vi "CDEW_SpecPage.vi"(10 "Spec Page Interface":T3, 11 "MetaDataObj in":refnum<class "MetaDataObj.lvclass">) -> (3 "MetaDataObj out":refnum<class "MetaDataObj.lvclass">)   [LabVIEW 2026, in "NIVS_CDEW_MetaDataObj.lvclass"]
uses:
  NIVS_CDEW_MetaDataObj.lvclass
  <resource>/dialog/NewProjectWizard/Spec Page Interface.ctl
  <resource>/dialog/NewProjectWizard/MetaDataObj/MetaDataObj.lvclass
  Types/Execution Modes.ctl
  Types/Wizard Conditional Controls.ctl
  NIVS_CDEW_MetaDataObj.lvclass/NIVS_CDEW_MetaDataObj.ctl
  <resource>/dialog/NewProjectWizard/MetaDataObj/MetaDataObj.lvclass/MetaDataObj.ctl
  <resource>/dialog/NewProjectWizard/MetaDataObj/Accessors/Write Project Name.vi
  <resource>/dialog/NewProjectWizard/MetaDataObj/Accessors/Write Project Root.vi
  C:/Program Files/National Instruments/LabVIEW 2026/resource/dialog/NewProjectWizard/MetaDataObj/MetaDataObj.lvclass
  C:/Program Files/National Instruments/LabVIEW 2026/ProjectTemplates/Source/NI VeriStand/Custom Device Express/Custom Device/NIVS_CDEW_MetaDataObj/NIVS_CDEW_MetaDataObj.lvclass
panel:
  out "error out":errorcluster
  out "Warning":string="*LabVIEW RT not installed, Linux_x64 disabled!"
  in  "Custom Device Target OS":enum16{"Linux_x64", "Windows", "All"}(ring)
  in  "Operation":T1(ring)
  in  "LaunchXMLEditor":bool
  in  "Custom Device Execution Mode":T2
  in  "Custom Device Name":string
  in  "Custom Device Root Folder":path=path "<specify path>"
  in  "Custom Device XML File":path=path "<specify path>"
  in  "Retain .Net APIs":bool
  in  "Retain LV Projects":bool
  in  "Parent Menu Name":string="National Instruments"
  in  "Submenu":bool
  in  "Maximum Custom Device Instances":i32=1 min=1 max=2474 step=1
  # "Advanced Options"
  # "Insert Custom Device in Submenu"
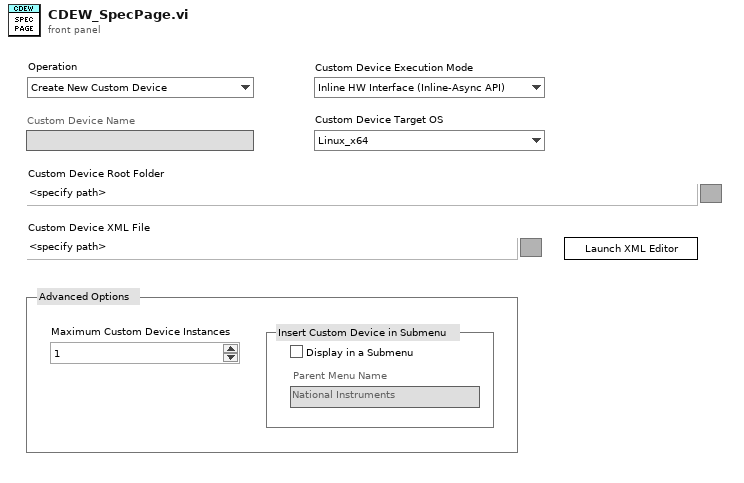
[diagram p1: front panel]
types:
  T1 = enum16{"Create New Custom Device", "Edit Existing Custom Device"}
  T2 = typedef "NIVS_CDEW_MetaDataObj.lvclass/Execution Modes.ctl" = enum16{"Inline HW Interface (Inline-Async API)", "Inline HW Interface"}
  T3 = typedef "Spec Page Interface.ctl" = cluster{"\"Tab Forward To\" Refnum":refnum<vi>, "\"Tab Backward To\" Refnum":refnum<vi>, "Errors":refnum<user-event>, "Quit":refnum<user-event>}
  T4 = typedef "NIVS_CDEW_MetaDataObj.lvclass/Wizard Conditional Controls.ctl" = cluster{"XML File Path":refnum<vi>, "Submenu":refnum<vi>, "Parent Menu Name":refnum<vi>, "Retain .Net APIs":refnum<vi>, "User Action":refnum<vi>, "Execution Mode":refnum<vi>}
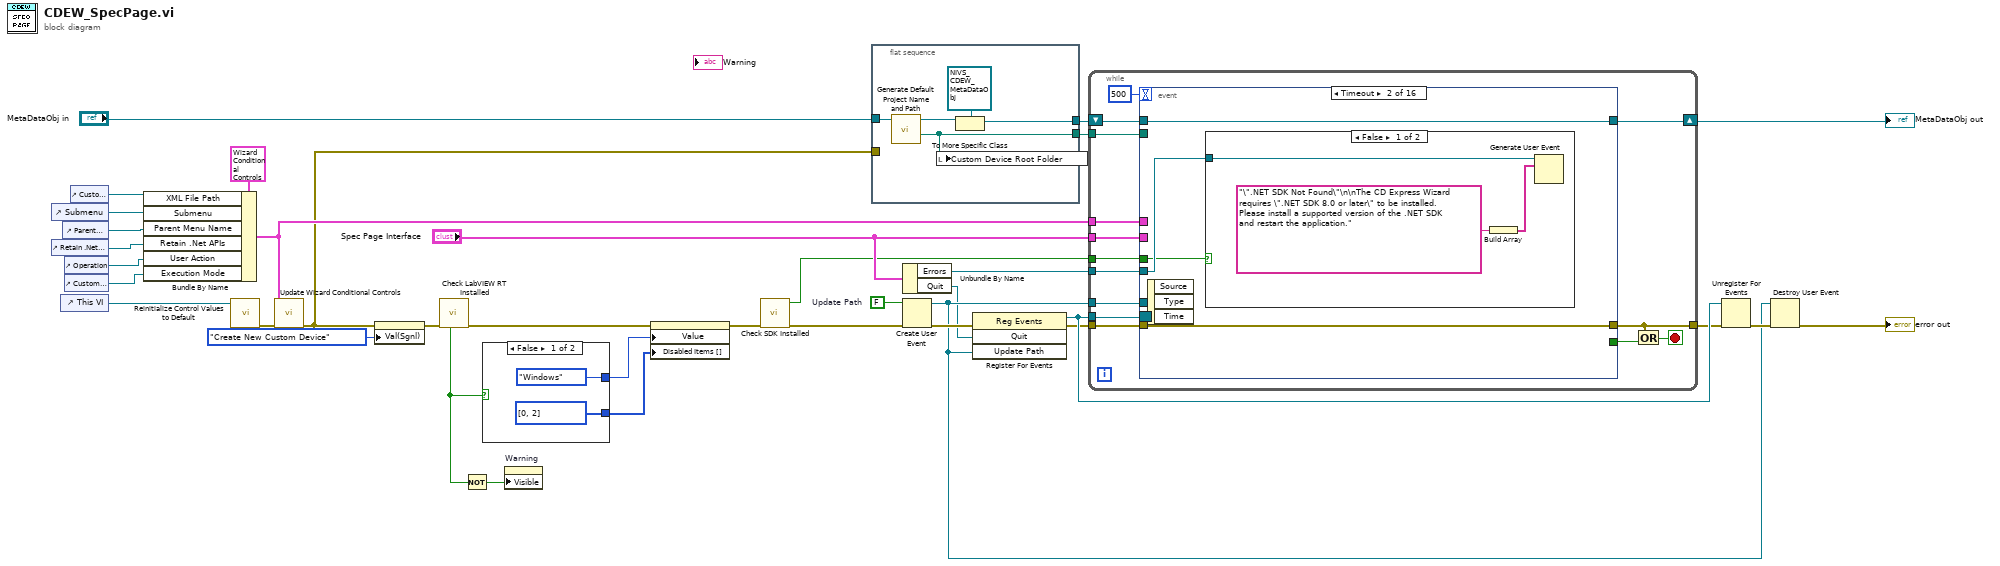
[diagram p0: block diagram]
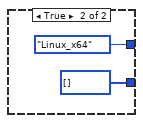
[diagram p2: hidden frame]
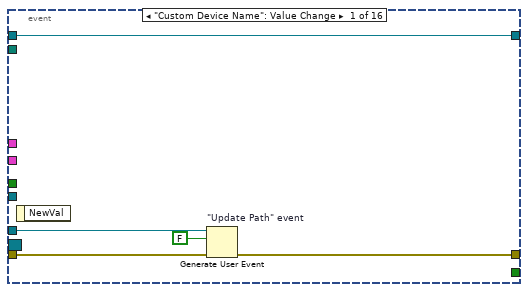
[diagram p3: hidden frame]
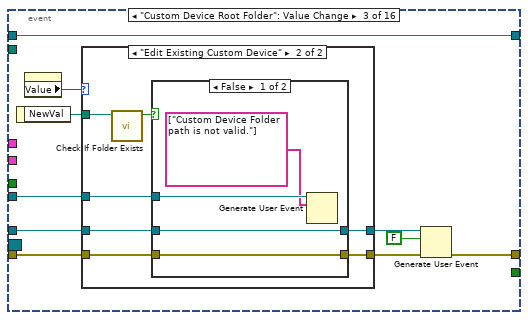
[diagram p5: hidden frame]
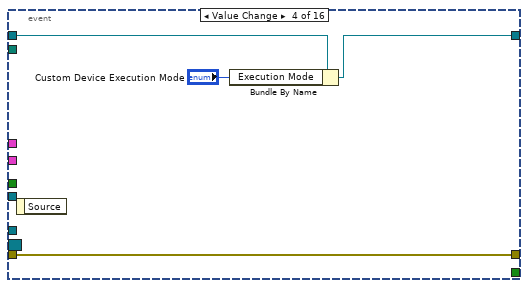
[diagram p8: hidden frame]
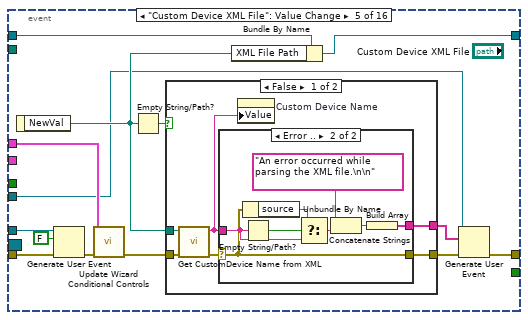
[diagram p9: hidden frame]
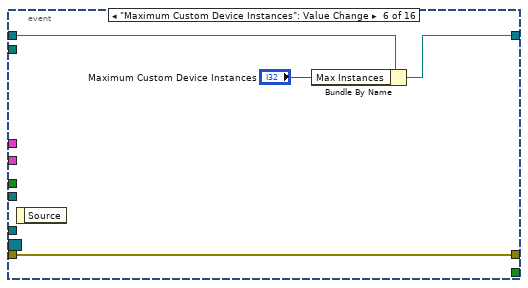
[diagram p12: hidden frame]
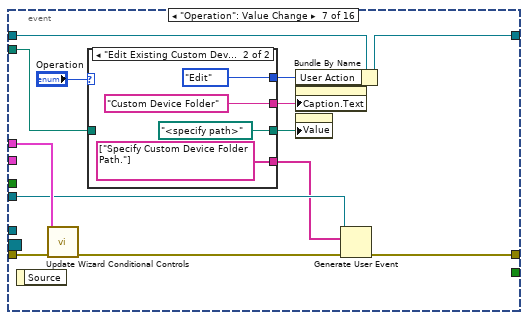
[diagram p13: hidden frame]
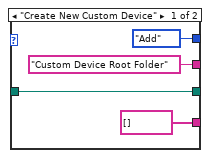
[diagram p14: hidden frame]
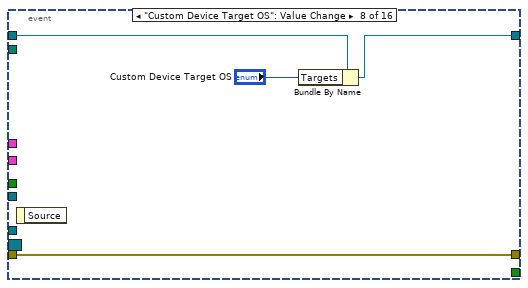
[diagram p15: hidden frame]
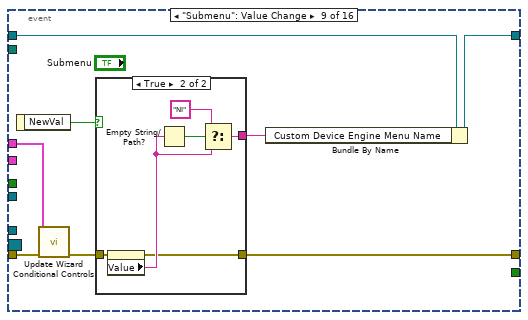
[diagram p16: hidden frame]
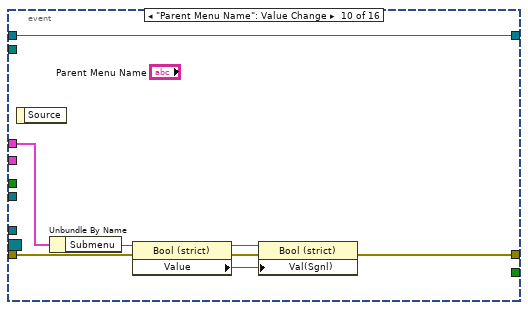
[diagram p18: hidden frame]
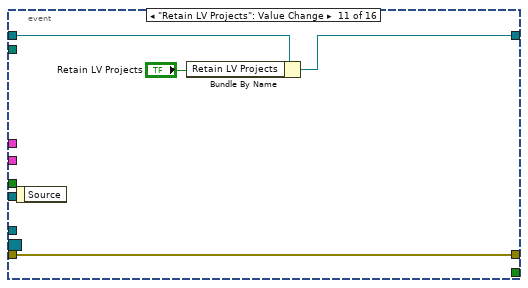
[diagram p19: hidden frame]
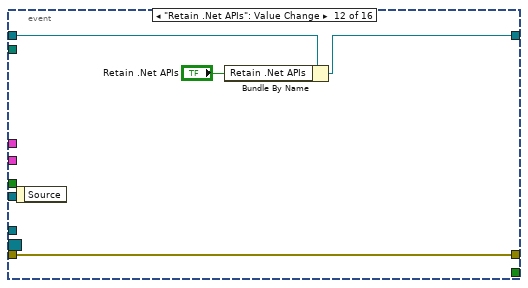
[diagram p20: hidden frame]
diagram:
  w19 = FALSE  # Update Path
  n1 = control-ref of="Submenu"() -> (w32:refnum<vi>)
  n2 = control-ref of="Retain .Net APIs"() -> (w34:refnum<vi>)
  n3 = control-ref of="This VI"() -> (w35:refnum<vi>)
  n4 = control-ref of="Parent Menu Name"() -> (w33:refnum<vi>)
  n5 = control-ref of="Operation"() -> (w25:refnum<vi>)
  n6 = control-ref of="Custom Device Execution Mode"() -> (w26:refnum<vi>)
  n7 = control-ref of="Custom Device XML File"() -> (w31:refnum<vi>)
  n8 = Bundle By Name(cluster=T4 {"XML File Path"=refnum, "Submenu"=refnum, "Parent Menu Name"=refnum, "Retain .Net APIs"=refnum, "User Action"=refnum, "Execution Mode"=refnum} ("Wizard_ConditionalControls"), "XML File Path"=w31, "Submenu"=w32, "Parent Menu Name"=w33, "Retain .Net APIs"=w34, "User Action"=w25, "Execution Mode"=w26) -> (w36:T4)
  n9 = call "Reinitialize Control Values to Default.vi"("VI Ref"=w35) -> ("error out"=w29:errorcluster)  [unwired: 10 in]
  n10 = call "Update Wizard Conditional Controls.vi"("error in"=w29, "Wizard_Conditional Controls"=w36) -> ("error out"=w24:errorcluster)  [unwired: 9 in]
  n11 = property on="Operation" class="Enum (strict)"(error in=w24, "Val(Sgnl)"=T1."Create New Custom Device" ("Value (Signaling)")) -> (error out=w7:errorcluster)  [unwired: 1 in, 1 out]
  n12 = call "Check LabVIEW RT Installed.vi"("error in"=w7) -> ("error out"=w13:errorcluster, "labview rt installed?"=w10:bool)  [unwired: 5 in, 4 out]
  n13 = Not(x=w10) -> (.not. x?=w9:bool)
  n14 = case shown="False" w10 {
    tunnel: [enum16{"Linux_x64", "Windows", "All"}."Windows" ("Custom Device Target OS") enum16{"Linux_x64", "Windows", "All"}."Linux_x64" ("Custom Device Target OS")] -> w12
    tunnel: [i32[] [0, 2] ("Disabled Items []") i32[] [] ("Disabled Items []")] -> w11
    frame False {
    }
    frame True {
    }
  }
  n15 = property on="Warning" class="Str"("Visible"=w9) -> ()  [unwired: 2 in, 2 out]
  n16 = property on="Custom Device Target OS" class="Enum (strict)"(error in=w13, "Value"=w12, "Disabled Items []"=w11) -> (error out=w3:errorcluster)  [unwired: 1 in, 1 out]
  n17 = call "Check SDK Installed.vi"("error in"=w3) -> ("error out"=w2:errorcluster, ".Net SDK Available?"=w1:bool)  [unwired: 9 in]
  n18 = flat-sequence {
    tunnel: [w44] -> w16
    tunnel: "MetaDataObj in" -> [w43]
    tunnel: w24 -> [_]
    tunnel: [w41] -> w14
    frame #0 {
      n19 = call <resource>:"Generate Default Project Name and Path.vi"("DNL_MetaDataObj in"=w43) -> ("Project Root"=w41:path, "DNL_MetaDataObj out"=w42:refnum<class "MetaDataObj.lvclass">)  [unwired: 8 in, 1 out]
      n20 = local write "Custom Device Root Folder"(w41) -> ()
      n21 = To More Specific Class(target class=refnum<class "NIVS_CDEW_MetaDataObj.lvclass"> refnum ("Consolidated_CD"), reference=w42) -> (specific class reference=w44:refnum<class "NIVS_CDEW_MetaDataObj.lvclass">)  [unwired: 1 in, 1 out]
    }
  }
  n22 = Unbundle By Name("Spec Page Interface") -> ("Errors"=w5:refnum<user-event>, "Quit"=w6:refnum<user-event>)
  n23 = Create User Event(user event datatype=w19, error in=w2) -> (user event=w15:refnum<user-event>, error out=w18:errorcluster)
  n24 = register-events(error in=w18, w6, w15) -> (reference out=w21:refnum<event-registration>, error out=w4:errorcluster)  [unwired: 1 in]
  n25 = while {
    tunnel: "Spec Page Interface" -> [w58]
    shift-right: [w57] -> w28
    shift-left: w16 -> [w56]
    tunnel: w21 -> [w59]
    tunnel: [w53] -> w20
    tunnel: w4 -> [w52]
    tunnel: w15 -> [w51]
    tunnel: w36 -> [w50]
    tunnel: w5 -> [w49]
    tunnel: w14 -> [w48]
    tunnel: w1 -> [w46]
    stop <- w55 stop-if-true
    n26 = event shown="[1] Timeout" {
      selector: w59 -> [_ _ _ _ _ _ _ _ _ _ _ _ _ _ _ _]
      dyn-events: _ -> [_ _ _ _ _ _ _ _ _ _ _ _ _ _ _ _]
      timeout: 500 -> [_ _ _ _ _ _ _ _ _ _ _ _ _ _ _ _]
      tunnel: w58 -> [_ _ _ _ _ _ _ _ _ _ _ _ _ w202 _ _]
      tunnel: [_ _ _ _ _ _ _ _ _ _ _ _ _ _ _ w220] -> w54
      tunnel: [w64 w66 w80 w100 w103 w134 w139 w159 w161 w176 w186 w190 w197 w198 w208 w217] -> w53
      tunnel: [w62 w68 w81 w98 w114 w132 w147 w158 w167 w178 w185 w188 w195 w199 w210 w219] -> w57
      tunnel: w56 -> [w62 w68 w81 w99 w113 w131 w146 w157 w166 w178 w184 w187 w194 w199 w209 w219]
      tunnel: w52 -> [w61 w66 w77 w100 w110 w134 w135 w159 w160 w175 w186 w190 w197 w198 w207 w216]
      tunnel: w51 -> [w60 _ w78 _ w109 _ _ _ _ _ _ _ _ _ _ _]
      tunnel: w50 -> [_ _ _ _ w112 _ w143 _ w163 w182 _ _ w193 _ _ _]
      tunnel: w49 -> [_ w67 w72 _ w102 _ w138 _ _ _ _ _ _ _ _ w218]
      tunnel: w48 -> [_ _ _ _ _ _ w140 _ _ _ _ _ _ _ _ _]
      tunnel: w46 -> [_ w65 _ _ _ _ _ _ _ _ _ _ _ _ _ _]
      event "Custom Device Name": Value Change {
        n27 = event-data() -> ()  [unwired: 1 in, 1 out]
        n28 = Generate User Event "\"Update Path\" event"(user event=w60, event data cluster=FALSE ("event data"), error in=w61) -> (error out=w64:errorcluster)  [unwired: 1 in, 1 out]
      }
      event Timeout {
        n29 = event-data() -> ()  [unwired: 1 in, 3 out]
        n30 = case shown="False" w65 {
          tunnel: w67 -> [w71 _]
          frame False {
            n31 = Build Array("\".NET SDK Not Found\"\n\nThe CD Express Wizard requires \".NET SDK 8.0 or later\" to be installed. Please install a supported version of the .NET SDK and restart the application." ("message")) -> (w69:string[])
            n32 = Generate User Event(user event=w71, event data cluster=w69) -> ()  [unwired: 2 in, 2 out]
          }
          frame True {
          }
        }
      }
      event "Custom Device Root Folder": Value Change {
        n33 = event-data() -> ("NewVal"=w73:path)  [unwired: 1 in]
        n34 = property on="Operation" class="Enum (strict)"() -> ("Value"=w76:T1)  [unwired: 2 in, 2 out]
        n35 = case shown="\"Edit Existing Custom Device\"" w76 {
          tunnel: w78 -> [w82 w88]
          tunnel: w77 -> [w83 w89]
          tunnel: [w83 w85] -> w75
          tunnel: [w82 w84] -> w74
          tunnel: w73 -> [_ w90]
          tunnel: w72 -> [_ w86]
          frame "Create New Custom Device" {
          }
          frame "Edit Existing Custom Device" {
            n36 = call "Check If Folder Exists.vi"("Folder Path"=w90) -> ("Valid Folder?"=w87:bool)  [unwired: 10 in]
            n37 = case shown="False" w87 {
              tunnel: w89 -> [w92 w96]
              tunnel: w88 -> [w93 w95]
              tunnel: w86 -> [w94 _]
              tunnel: [w92 w96] -> w85
              tunnel: [w93 w95] -> w84
              frame False {
                n38 = Generate User Event ("\"Update Path\" event")(user event=w94, event data cluster=string[] ["Custom Device Folder path is not valid."] ("event data")) -> ()  [unwired: 2 in, 2 out]
              }
              frame True {
              }
            }
          }
        }
        n39 = Generate User Event ("\"Update Path\" event")(user event=w74, event data cluster=FALSE ("event data"), error in=w75) -> (error out=w80:errorcluster)  [unwired: 1 in, 1 out]
      }
      event Value Change {
        n40 = event-data() -> ()  [unwired: 1 in, 1 out]
        n41 = Bundle By Name(cluster=w99, "Execution Mode"="Custom Device Execution Mode") -> (w98:refnum<class "NIVS_CDEW_MetaDataObj.lvclass">)
      }
      event "Custom Device XML File": Value Change {
        n42 = event-data() -> ("NewVal"=w105:path)  [unwired: 1 in]
        n43 = Generate User Event ("\"Update Path\" event")(user event=w109, event data cluster=FALSE ("event data"), error in=w110) -> (error out=w108:errorcluster)  [unwired: 1 in, 1 out]
        n44 = call "Update Wizard Conditional Controls.vi"("error in"=w108, "Wizard_Conditional Controls"=w112) -> ("error out"=w107:errorcluster)  [unwired: 9 in]
        n45 = Empty String/Path?(string/path=w105) -> (empty?=w106:bool)
        n46 = case shown="False" w106 {
          tunnel: w107 -> [w120 w130]
          tunnel: w105 -> [w119 _]
          tunnel: [w117 w130] -> w104
          tunnel: [w116 _] -> w101
          frame False {
            n47 = call "Get CustomDevice Name from XML.vi"("error in"=w120, "XML File Path"=w119) -> ("error out"=w118:errorcluster, "Custom Device Name"=w115:string)  [unwired: 8 in]
            n48 = case shown="Error .." w118 {
              selector: w118 -> [w121 w122]
              tunnel: w115 -> [_ w128]
              tunnel: [_ w123] -> w116
              tunnel: [w121 w122] -> w117
              frame No Error {
              }
              frame Error {
                n49 = Unbundle By Name(w122) -> ("source"=w127:string)
                n50 = Empty String/Path?(string/path=w128) -> (empty?=w129:bool)
                n51 = Select(t=w127, s=w129, f=w128) -> (s? t:f=w126:string)
                n52 = Concatenate Strings("An error occurred while parsing the XML file.\n\n" ("string"), w126) -> (w124:string)
                n53 = Build Array(w124) -> (w123:string[])
              }
            }
            n54 = property on="Custom Device Name" class="Str"("Value"=w115) -> ()  [unwired: 2 in, 2 out]
          }
          frame True {
          }
        }
        n55 = Bundle By Name(cluster=w113, "XML File Path"=w105) -> (w114:refnum<class "NIVS_CDEW_MetaDataObj.lvclass">)
        n56 = Generate User Event ("\"Update Path\" event")(user event=w102, event data cluster=w101, error in=w104) -> (error out=w103:errorcluster)  [unwired: 1 in, 1 out]
      }
      event "Maximum Custom Device Instances": Value Change {
        n57 = event-data() -> ()  [unwired: 1 in, 1 out]
        n58 = Bundle By Name(cluster=w131, "Max Instances"="Maximum Custom Device Instances") -> (w132:refnum<class "NIVS_CDEW_MetaDataObj.lvclass">)
      }
      event "Operation": Value Change {
        n59 = event-data() -> ()  [unwired: 1 in, 1 out]
        n60 = call "Update Wizard Conditional Controls.vi"("error in"=w135, "Wizard_Conditional Controls"=w143) -> ("error out"=w136:errorcluster)  [unwired: 9 in]
        n61 = case shown="\"Edit Existing Custom Device\"" "Operation" {
          tunnel: [enum16{"Add", "Edit"}."Add" ("User Action") enum16{"Add", "Edit"}."Edit" ("User Action")] -> w144
          tunnel: ["Custom Device Root Folder" "Custom Device Folder"] -> w142
          tunnel: [w149 path "<specify path>"] -> w141
          tunnel: w140 -> [w149 _]
          tunnel: [string[] [] ("event data") string[] ["Specify Custom Device Folder Path."] ("event data")] -> w137
          frame "Create New Custom Device" {
          }
          frame "Edit Existing Custom Device" {
          }
        }
        n62 = Bundle By Name(cluster=w146, "User Action"=w144) -> (w147:refnum<class "NIVS_CDEW_MetaDataObj.lvclass">)
        n63 = property on="Custom Device Root Folder" class="Path"("Caption.Text"=w142) -> ()  [unwired: 2 in, 2 out]
        n64 = property on="Custom Device Root Folder" class="Path"("Value"=w141) -> ()  [unwired: 2 in, 2 out]
        n65 = Generate User Event(user event=w138, event data cluster=w137, error in=w136) -> (error out=w139:errorcluster)  [unwired: 1 in, 1 out]
      }
      event "Custom Device Target OS": Value Change {
        n66 = event-data() -> ()  [unwired: 1 in, 1 out]
        n67 = Bundle By Name(cluster=w157, "Targets"="Custom Device Target OS") -> (w158:refnum<class "NIVS_CDEW_MetaDataObj.lvclass">)
      }
      event "Submenu": Value Change {
        n68 = event-data() -> ("NewVal"=w165:bool)  [unwired: 1 in]
        n69 = call "Update Wizard Conditional Controls.vi"("error in"=w160, "Wizard_Conditional Controls"=w163) -> ("error out"=w162:errorcluster)  [unwired: 9 in]
        n70 = case shown="True" w165 {
          tunnel: [_ w171] -> w164
          tunnel: w162 -> [w168 w170]
          tunnel: [w168 w169] -> w161
          frame False {
          }
          frame True {
            n71 = property on="Parent Menu Name" class="Str"(error in=w170) -> (error out=w169:errorcluster, "Value"=w172:string)  [unwired: 1 in, 1 out]
            n72 = Empty String/Path?(string/path=w172) -> (empty?=w174:bool)
            n73 = Select(t="NI", s=w174, f=w172) -> (s? t:f=w171:string)
          }
        }
        n74 = Bundle By Name(cluster=w166, "Custom Device Engine Menu Name"=w164) -> (w167:refnum<class "NIVS_CDEW_MetaDataObj.lvclass">)
      }
      event "Parent Menu Name": Value Change {
        n75 = event-data() -> ()  [unwired: 1 in, 1 out]
        n76 = Unbundle By Name(w182) -> ("Submenu"=w181:refnum<vi>)
        n77 = property class="Bool (strict)"(reference=w181, error in=w175) -> (reference out=w180:refnum<vi>, error out=w177:errorcluster, "Value"=w179:bool)
        n78 = property class="Bool (strict)"(reference=w180, error in=w177, "Val(Sgnl)"=w179) -> (error out=w176:errorcluster)  [unwired: 1 out]
      }
      event "Retain LV Projects": Value Change {
        n79 = event-data() -> ()  [unwired: 1 in, 1 out]
        n80 = Bundle By Name(cluster=w184, "Retain LV Projects"="Retain LV Projects") -> (w185:refnum<class "NIVS_CDEW_MetaDataObj.lvclass">)
      }
      event "Retain .Net APIs": Value Change {
        n81 = event-data() -> ()  [unwired: 1 in, 1 out]
        n82 = Bundle By Name(cluster=w187, "Retain .Net APIs"="Retain .Net APIs") -> (w188:refnum<class "NIVS_CDEW_MetaDataObj.lvclass">)
      }
      event "LaunchXMLEditor": Value Change {
        n83 = event-data() -> ()  [unwired: 1 in, 1 out]
        n84 = Unbundle By Name(w193) -> ("XML File Path"=w192:refnum<vi>)
        n85 = Unbundle By Name(w194) -> ("XML File Path"=w196:path)
        n86 = call "Main UI.vi"("XML File"=w196) -> ("Selected XML File"=w191:path)  [unwired: 10 in]
        n87 = Bundle By Name(cluster=w194, "XML File Path"=w191) -> (w195:refnum<class "NIVS_CDEW_MetaDataObj.lvclass">)
        n88 = property class="Path"(reference=w192, "Val(Sgnl)"=w191) -> ()  [unwired: 1 in, 2 out]
      }
      event Key Down? {
        n89 = event-data() -> ("Char"=w205:i16, "PlatMods.Shift"=w204:bool)  [unwired: 1 in]
        n90 = Unbundle By Name(w202) -> ("\"Tab Forward To\" Refnum"=w201:refnum<vi>, "\"Tab Backward To\" Refnum"=w200:refnum<vi>)
        n91 = control-ref of="Custom Device Name"() -> (w203:refnum<vi>)
        n92 = call <resource>:"HandleInnerVITabbing.vi"("Tab Backward To"=w200, "Tab Forward To"=w201, "Char"=w205, "First Control"=w203, "Shift"=w204) -> ("Discard"=w206:bool)  [unwired: 6 in]
        n93 = event-data("Discard?"=w206) -> ()  [unwired: 1 in, 1 out]
      }
      event User Event {
        n94 = event-data() -> ()  [unwired: 1 in, 1 out]
        n95 = property class="Consolidated_CD"(reference=w209, error in=w207, "Project Name"="Custom Device Name", "Project Root"="Custom Device Root Folder") -> (reference out=w210:refnum<class "NIVS_CDEW_MetaDataObj.lvclass">, error out=w208:errorcluster)
      }
      event User Event {
        w220 = TRUE  # Quit
        n96 = event-data() -> ()  [unwired: 1 in, 1 out]
        n97 = property on="Custom Device XML File" class="Path"() -> ("Value"=w215:path)  [unwired: 2 in, 2 out]
        n98 = Empty String/Path?(string/path=w215) -> (empty?=w214:bool)
        n99 = case shown="True" w214 {
          tunnel: w218 -> [_ w225]
          tunnel: [w221 w224] -> w217
          tunnel: w216 -> [w221 w223]
          tunnel: string[] ["XML File path cannot be Empty "] ("event data") -> [_ w222]
          frame False {
          }
          frame True {
            n100 = Generate User Event(user event=w225, event data cluster=w222, error in=w223) -> (error out=w224:errorcluster)  [unwired: 1 in, 1 out]
          }
        }
      }
    }
    n101 = Or(x=w53, y=w54) -> (x .or. y?=w55:bool)
  }
  "MetaDataObj out" <- w28
  n102 = Unregister For Events(event registration refnum=w21, error in=w20) -> (error out=w17:errorcluster)
  n103 = Destroy User Event(user event=w15, error in=w17) -> (error out=→"error out":errorcluster)
